vi "multiple_consumer.vi"() -> ()   [LabVIEW 2020]
uses:
  Type Defs/Message.ctl
panel:
  in  "Stop Button":bool
  in  "Start Button":bool
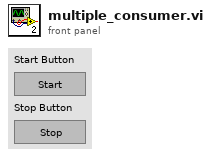
[diagram p1: front panel]
types:
  T1 = typedef "Message.ctl" = cluster{"Command":string, "Data":variant}
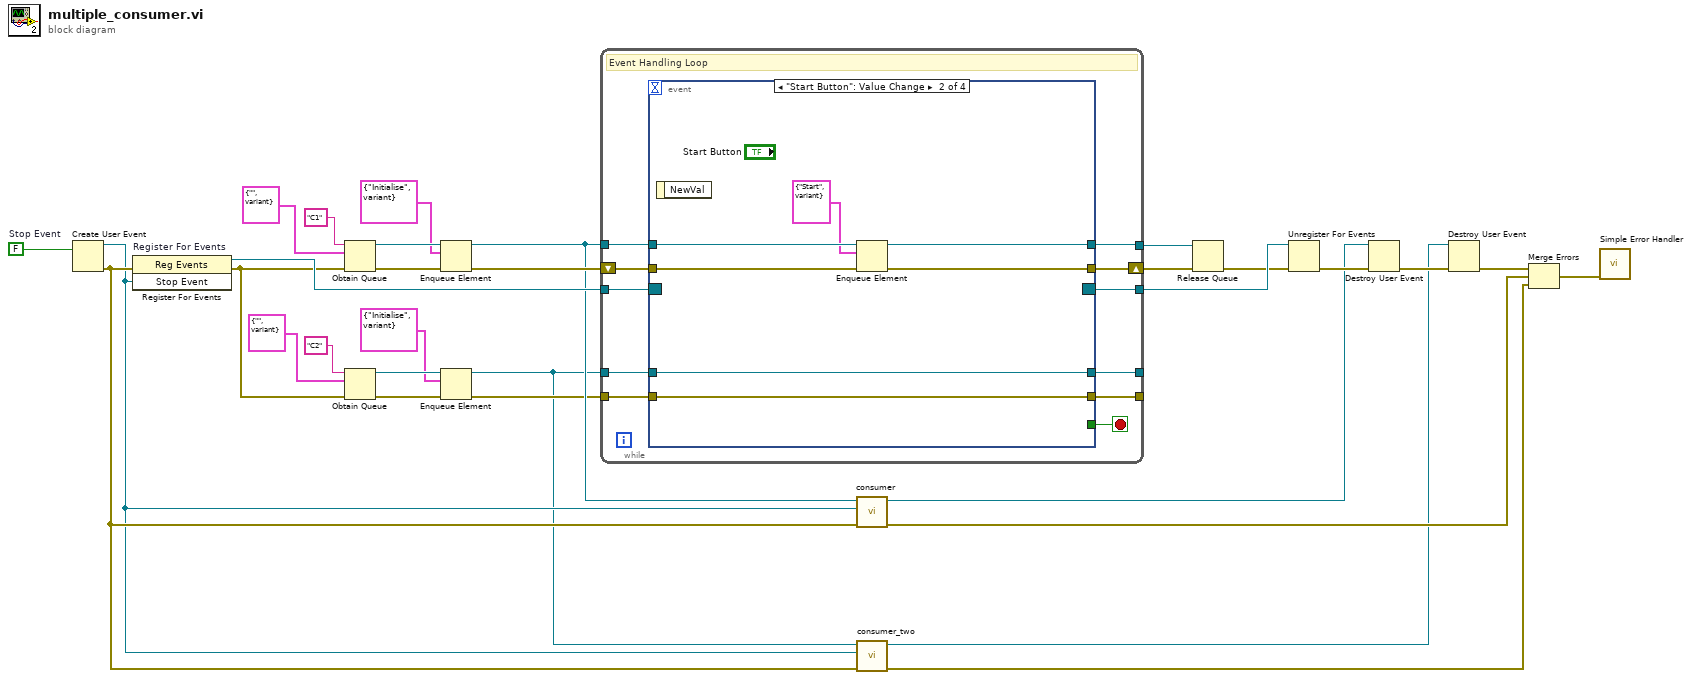
[diagram p0: block diagram]
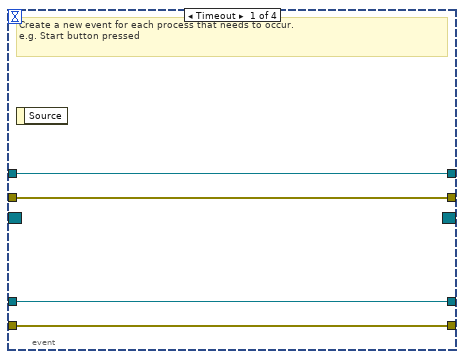
[diagram p2: hidden frame]
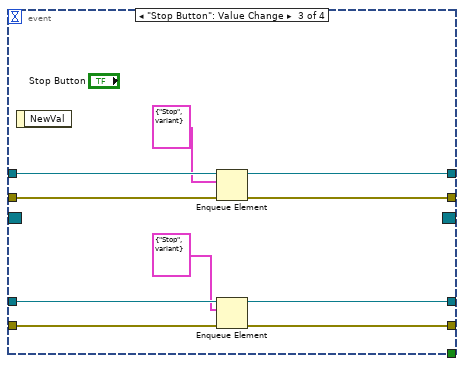
[diagram p3: hidden frame]
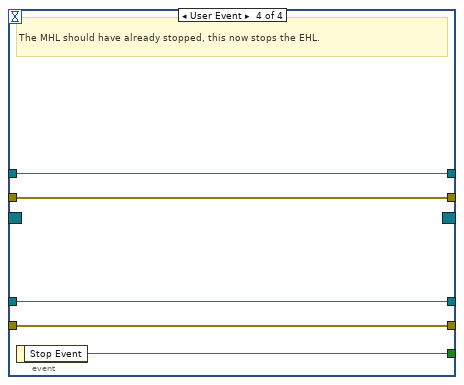
[diagram p4: hidden frame]
diagram:
  w17 = FALSE  # Stop Event
  n1 = Create User Event(user event datatype=w17) -> (user event=w15:refnum<user-event>, error out=w16:errorcluster)  [unwired: 1 in]
  n2 = register-events "Register For Events"(error in=w16, w15) -> (reference out=w28:refnum<event-registration>, error out=w10:errorcluster)  [unwired: 1 in]
  n3 = Obtain Queue(name (unnamed)="C1", element data type=T1 {"Command"="", "Data"=variant} ("Consumer1"), error in (no error)=w10) -> (queue out=w22:refnum<queue>, error out=w21:errorcluster)  [unwired: 2 in, 1 out]
  n4 = Obtain Queue(name (unnamed)="C2", element data type=T1 {"Command"="", "Data"=variant} ("Consumer2"), error in (no error)=w10) -> (queue out=w12:refnum<queue>, error out=w13:errorcluster)  [unwired: 2 in, 1 out]
  n5 = Enqueue Element(queue=w22, element=T1 {"Command"="Initialise", "Data"=variant}, error in (no error)=w21) -> (queue out=w19:refnum<queue>, error out=w20:errorcluster)  [unwired: 1 in, 1 out]
  n6 = Enqueue Element(queue=w12, element=T1 {"Command"="Initialise", "Data"=variant}, error in (no error)=w13) -> (queue out=w6:refnum<queue>, error out=w9:errorcluster)  [unwired: 1 in, 1 out]
  n7 = while {
    tunnel: w19 -> [w40]
    shift-right: [w41] -> w29
    shift-left: w20 -> [w42]
    tunnel: [w39] -> w30
    tunnel: w28 -> [w38]
    tunnel: [w37] -> w27
    tunnel: w9 -> [w35]
    tunnel: w6 -> [w33]
    tunnel: [w34] -> _
    tunnel: [w32] -> _
    stop <- w36 stop-if-true
    # "Event Handling Loop"
    n8 = event shown="[1] \"Start Button\": Value Change" {
      selector: w38 -> [_ _ _ _]
      dyn-events: [_ _ _ _] -> w37
      timeout: _ -> [_ _ _ _]
      tunnel: w42 -> [w46 w53 w63 w68]
      tunnel: [w46 w52 w62 w68] -> w41
      tunnel: w40 -> [w45 w51 w61 w67]
      tunnel: [w45 w50 w60 w67] -> w39
      tunnel: [_ _ _ w66] -> w36
      tunnel: w35 -> [w44 w48 w58 w65]
      tunnel: [w44 w48 w57 w65] -> w34
      tunnel: w33 -> [w43 w47 w56 w64]
      tunnel: [w43 w47 w55 w64] -> w32
      event Timeout {
        # "Create a new event for each process that needs to occur. \ne.g. Start button pressed"
        n9 = event-data() -> ()  [unwired: 1 in, 1 out]
      }
      event "Start Button": Value Change {
        n10 = event-data() -> ()  [unwired: 1 in, 1 out]
        n11 = Enqueue Element(queue=w51, element=T1 {"Command"="Start", "Data"=variant}, error in (no error)=w53) -> (queue out=w50:refnum<queue>, error out=w52:errorcluster)  [unwired: 1 in, 1 out]
      }
      event "Stop Button": Value Change {
        n12 = event-data() -> ()  [unwired: 1 in, 1 out]
        n13 = Enqueue Element(queue=w61, element=T1 {"Command"="Stop", "Data"=variant}, error in (no error)=w63) -> (queue out=w60:refnum<queue>, error out=w62:errorcluster)  [unwired: 1 in, 1 out]
        n14 = Enqueue Element(queue=w56, element=T1 {"Command"="Stop", "Data"=variant}, error in (no error)=w58) -> (queue out=w55:refnum<queue>, error out=w57:errorcluster)  [unwired: 1 in, 1 out]
      }
      event User Event {
        # "The MHL should have already stopped, this now stops the EHL."
        n15 = event-data() -> ("Stop Event"=w66:bool)  [unwired: 1 in]
      }
    }
  }
  n16 = call "consumer.vi"("error in (no error)"=w16, "Stop Event in"=w15, "Queue in"=w19) -> ("error out"=w24:errorcluster, "User Event out"=w4:refnum<user-event>)  [unwired: 7 in]
  n17 = call "consumer_two.vi"("error in (no error)"=w16, "Stop Event in"=w15, "Queue in"=w6) -> ("error out"=w5:errorcluster, "User Event out"=w1:refnum<user-event>)  [unwired: 7 in]
  n18 = Release Queue(queue=w30, error in (no error)=w29) -> (error out=w25:errorcluster)  [unwired: 1 in, 2 out]
  n19 = Unregister For Events(event registration refnum=w27, error in=w25) -> (error out=w26:errorcluster)
  n20 = Destroy User Event(user event=w4, error in=w26) -> (error out=w3:errorcluster)
  n21 = Destroy User Event(user event=w1, error in=w3) -> (error out=w2:errorcluster)
  n22 = Merge Errors(w2, w24, w5) -> (w23:errorcluster)
  n23 = call <vilib>:"Simple Error Handler.vi"("error in (no error)"=w23) -> ()  [unwired: 4 in, 5 out]
